vi "Replicate.vi"(2 "stream":T1, 3 "independent aborts? (F)":bool, 4 "copy 1 size (unlimited)":i32, 8 "copy 2 size (unlimited)":i32) -> (7 "stream copy 1":T1, 9 "stream copy 2":T1)   [LabVIEW 2017, in "Stream-t'WPI_EncoderType.ctl'.lvlib"]
doc: "Splits a Stream channel into two Stream channels so that each of the readers of the channels receives a separate copy of the data written into the original channel."
uses:
  <extravilib>/ChannelInstances/Stream-t'WPI_EncoderType.ctl'.lvlib
  <extravilib>/ChannelInstances/Stream-t'WPI_EncoderType.ctl'/)Channel.ctl
  <vilib>/Rock Robotics/WPI/Encoder/WPI_EncoderType.ctl
  <extravilib>/ChannelInstances/Stream-t'WPI_EncoderType.ctl'/EndpointRead.vi
  <extravilib>/ChannelInstances/Stream-t'WPI_EncoderType.ctl'/Endpoint.vi
  <extravilib>/ChannelInstances/Stream-t'WPI_EncoderType.ctl'/)Channel.vi
  <resource>/ChannelSupport/_ChannelSupport/WaitIfNeeded.vi
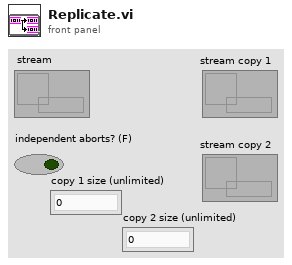
[diagram p1: front panel]
types:
  T1 = typedef "Stream-t'WPI_EncoderType.ctl'.lvlib/)Channel.ctl" = refnum<queue>
  T2 = typedef "WPI_EncoderType.ctl" = enum16{"1x", "2x", "4x"}
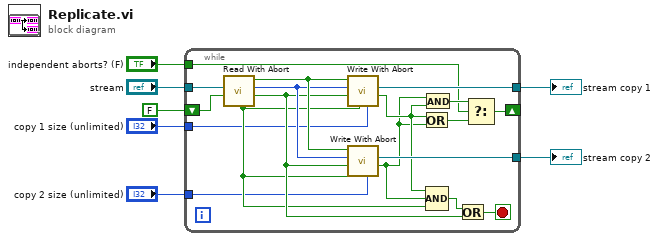
[diagram p0: block diagram]
diagram:
  n1 = while {
    tunnel: "stream" -> [w25]
    tunnel: [w21] -> w6
    tunnel: [w20] -> w5
    shift-right: [w9] -> _
    shift-left: FALSE -> [w22]
    tunnel: "copy 1 size (unlimited)" -> [w14]
    tunnel: "copy 2 size (unlimited)" -> [w15]
    tunnel: "independent aborts? (F)" -> [w8]
    stop <- w24 stop-if-true
    n2 = call <extravilib>:"Read With Abort.vi"("abort"=w22, "channel"=w25) -> ("last element?"=w17:bool, "element"=w18:T2, "element valid?"=w19:bool, "aborted?"=w16:bool)  [unwired: 4 in, 2 out]
    n3 = call <extravilib>:"Write With Abort.vi"("size (unlimited)"=w14, "abort"=w16, "last element? (F)"=w17, "element"=w18, "element valid? (T)"=w19) -> ("aborted?"=w13:bool, "channel"=w21:T1)  [unwired: 3 in, 2 out]
    n4 = call <extravilib>:"Write With Abort.vi"("size (unlimited)"=w15, "abort"=w16, "last element? (F)"=w17, "element"=w18, "element valid? (T)"=w19) -> ("aborted?"=w12:bool, "channel"=w20:T1)  [unwired: 3 in, 2 out]
    n5 = Or(x=w13, y=w12) -> (x .or. y?=w10:bool)
    n6 = And(x=w12, y=w13) -> (x .and. y?=w11:bool)
    n7 = Compound Arithmetic op=AND(w13, w12, w16) -> (w23:bool)
    n8 = Or(x=w23, y=w17) -> (x .or. y?=w24:bool)
    n9 = Select(t=w11, s=w8, f=w10) -> (s? t:f=w9:bool)
  }
  "stream copy 1" <- w6
  "stream copy 2" <- w5
